vi "Update Mapped Channels.vi"(8 "error in (no error)":errorcluster, 11 "Output Sequencer in":refnum<class "Output Sequencer.lvclass">) -> (0 "error out":errorcluster, 3 "Output Sequencer out":refnum<class "Output Sequencer.lvclass">)   [LabVIEW 2024, in "Output Sequencer.lvlib" / "Output Sequencer.lvclass"]
uses:
  Output Sequencer.lvclass
  C:/Program Files/National Instruments/LabVIEW 2024/vi.lib/FlexLogger/SDK/PluginSDK.lvlibp/PEFClasses/SDK/Plugin/Plugin.lvclass
  Types/UI Event.ctl
  Types/Event Type.ctl
  Output Sequencer.lvclass/Output Sequencer.ctl
  Globals/Global Strings.vi
  <vilib>/FlexLogger/SDK/PluginSDK.lvlibp/PEFClasses/SDK/Plugin/ParameterAccess/Read N Digital Channels.vi
  <vilib>/FlexLogger/SDK/PluginSDK.lvlibp/PEFClasses/SDK/Plugin/ParameterAccess/Read N Channel.vi
  <vilib>/FlexLogger/SDK/PluginSDK.lvlibp/PEFClasses/SDK/Plugin/Plugin.lvclass
  C:/Program Files/National Instruments/LabVIEW 2024/vi.lib/FlexLogger/SDK/PluginSDK.lvlibp/PEFClasses/SDK/Processing Element/Processing Element.lvclass
  C:/Dev/GitHub/ni/niflexlogger-plugins/PDK plugins/Output Sequencer/source/Output Sequencer/Output Sequencer.lvclass
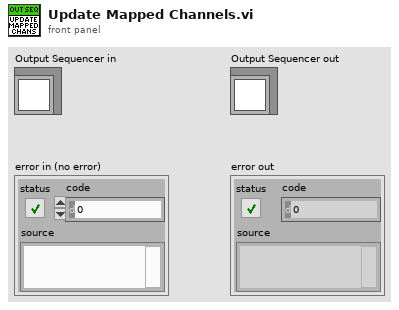
[diagram p1: front panel]
types:
  T1 = typedef "Output Sequencer.lvlib/Output Sequencer.lvclass/Event Type.ctl" = enum16{"Channel Update", "Test State Change", "Stop"}
  T2 = typedef "Output Sequencer.lvlib/Output Sequencer.lvclass/UI Event.ctl" = cluster{"Type":T1, "Data":variant}
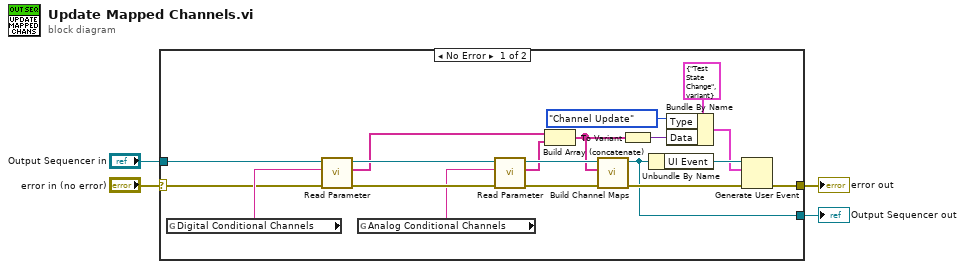
[diagram p0: block diagram]
diagram:
  n1 = case shown="No Error" "error in (no error)" {
    selector: "error in (no error)" -> [w5 w25]
    tunnel: "Output Sequencer in" -> [w19 w24]
    tunnel: [w10 w24] -> w3
    tunnel: [w9 w25] -> w2
    frame No Error {
      n2 = global read "Global Strings.vi" "Digital Conditional Channels"() -> (w20:string)
      n3 = call-poly <vilib>:"Read Parameter.vi"("error in (no error)"=w5, "Name (Unique Channel Identifier)"=w20, "Plugin in"=w19) -> ("error out"=w23:errorcluster, "Channels"=w8:string[], "Plugin out"=w22:refnum<class "Output Sequencer.lvclass">)  [unwired: 5 in, 1 out]
      n4 = global read "Global Strings.vi" "Analog Conditional Channels"() -> (w21:string)
      n5 = call-poly <vilib>:"Read Parameter.vi"("error in (no error)"=w23, "Name (Unique Channel Identifier)"=w21, "Plugin in"=w22) -> ("error out"=w12:errorcluster, "Channels"=w7:string[], "Plugin out"=w13:refnum<class "Output Sequencer.lvclass">)  [unwired: 5 in, 1 out]
      n6 = Build Array (concatenate)(w8, w7) -> (w6:string[])
      n7 = call "Build Channel Maps.vi"("error in (no error)"=w12, "Channels"=w6, "Output Sequencer in"=w13) -> ("error out"=w11:errorcluster, "Output Sequencer out"=w10:refnum<class "Output Sequencer.lvclass">)  [unwired: 7 in]
      n8 = To Variant(anything=w6) -> (Variant=w16:variant)
      n9 = Unbundle By Name(w10) -> ("UI Event"=w18:refnum<user-event>)
      n10 = Bundle By Name(cluster=T2 {"Type"=enum."Test State Change", "Data"=variant} ("event data"), "Type"=Event_Type."Channel Update", "Data"=w16) -> (w14:T2)
      n11 = Generate User Event(user event=w18, event data cluster=w14, error in=w11) -> (error out=w9:errorcluster)  [unwired: 1 in, 1 out]
    }
    frame Error {
    }
  }
  "Output Sequencer out" <- w3
  "error out" <- w2
